vi "Get Key Names.vi"(7 "Section":string, 8 "error in (no error)":errorcluster) -> (0 "error out":errorcluster, 2 "Keys":string[](array[string]))   [LabVIEW 2020, in "Configuration Manager.lvclass"]
uses:
  Configuration Manager.lvclass
  <vilib>/Utility/config.llb/NI_LVConfig.lvlib
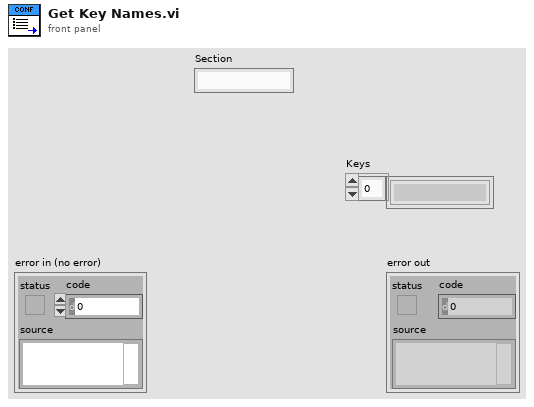
[diagram p1: front panel]
types:
  T1 = typedef "NI_LVConfig.lvlib/Config Data RefNum.ctl" = refnum<k1>
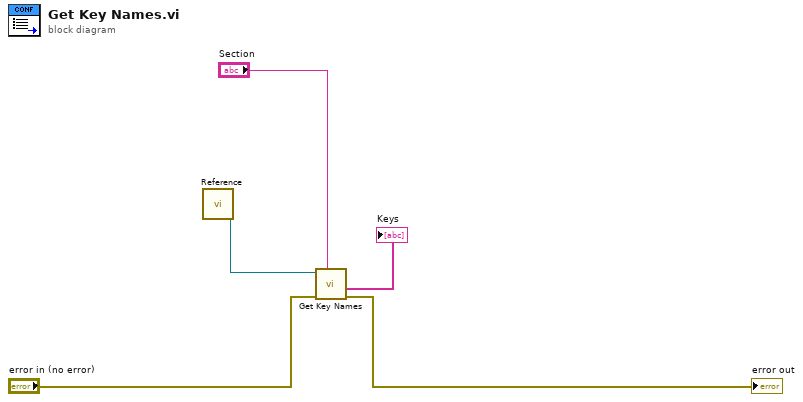
[diagram p0: block diagram]
diagram:
  n1 = call "Reference.vi"() -> ("Refnum out"=w5:T1)  [unwired: 10 in, 1 out]
  n2 = call <vilib>:"Get Key Names.vi"("section"="Section", "error in (no error)"="error in (no error)", "refnum"=w5) -> ("error out"=→"error out":errorcluster, "key names"=→"Keys":string[])  [unwired: 5 in, 2 out]
